vi "TestHTTP.vi"() -> ()   [LabVIEW 2025, in "MCP Server.lvlib"]
uses:
  MCP Server.lvlib
  MCP Handler/MCP Handler.lvclass
  C:/Program Files/National Instruments/LabVIEW 2025/vi.lib/IlluminatedG/IG HTTP Server/HTTP Server/Handler/Handler.lvclass
  <vilib>/IlluminatedG/IG HTTP Server/HTTP Server/Server/Add Connection Handler.vi
  <vilib>/IlluminatedG/IG HTTP Server/HTTP Server/Server/Add Request Handler.vi
  <vilib>/IlluminatedG/IG HTTP Server/HTTP Server/Server/Add Route Handler.vi
  <vilib>/IlluminatedG/IG HTTP Server/HTTP Server/Server/Add Controller Handler.vi
  <vilib>/IlluminatedG/IG HTTP Server/HTTP Server/Server/Add Controller.vi
  <vilib>/IlluminatedG/IG HTTP Server/HTTP Server/Server/Add Response Handler.vi
  <vilib>/IlluminatedG/IG HTTP Server/HTTP Server/Server/Add Complete Handler.vi
  <vilib>/IlluminatedG/IG HTTP Server/HTTP Server/Server/Add Exception Handler.vi
  <vilib>/IlluminatedG/IG HTTP Server/HTTP Server/Connection Handler/Connection Handler.lvclass
  <vilib>/IlluminatedG/IG HTTP Server/HTTP Server/Request Handler/Request Handler.lvclass
  <vilib>/IlluminatedG/IG HTTP Server/HTTP Server/Route Handler/Route Handler.lvclass
  <vilib>/IlluminatedG/IG HTTP Server/HTTP Server/Controller Handler/Controller Handler.lvclass
  <vilib>/IlluminatedG/IG HTTP Server/HTTP Server/Controller/Controller.lvclass
  <vilib>/IlluminatedG/IG HTTP Server/HTTP Server/Response Handler/Response Handler.lvclass
  <vilib>/IlluminatedG/IG HTTP Server/HTTP Server/Complete Handler/Complete Handler.lvclass
  <vilib>/IlluminatedG/IG HTTP Server/HTTP Server/Exception Handler/Exception Handler.lvclass
  <vilib>/IlluminatedG/IG HTTP Server/HTTP Server/Handler/Handler.lvclass
  C:/Program Files/National Instruments/LabVIEW 2025/vi.lib/IlluminatedG/IG HTTP Server/HTTP Server/Controller/Controller.lvclass
  C:/Users/jgoebel/OneDrive - Emerson/Dokumente/Praesentationen/MCP in LabVIEW/LabVIEW-MCP-Server-Toolkit/src/MCP Server/MCP Handler/MCP Handler.lvclass
  <vilib>/IlluminatedG/IG HTTP Server/HTTP Server/Server/Server.lvclass
panel:
  out "Numeric":i32
  in  "stop":bool
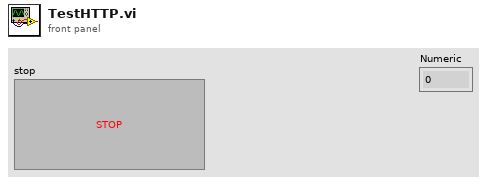
[diagram p1: front panel]
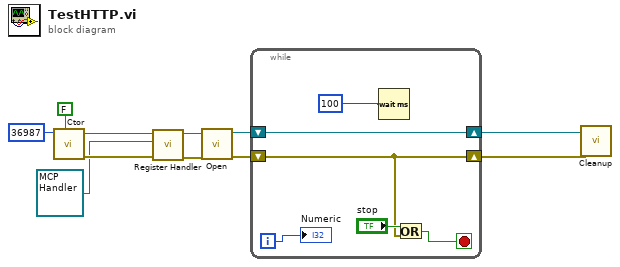
[diagram p0: block diagram]
diagram:
  n1 = call <vilib>:"Ctor.vi"("Debug (F)"=FALSE, "HTTP Port (80)"=u16 36987) -> ("error out"=w10:errorcluster, "Server out"=w11:refnum<class "Server.lvclass">)  [unwired: 8 in]
  n2 = call <vilib>:"Register Handler.vi"("error in (no error)"=w10, "Handler"=refnum<class "MCP Handler.lvclass"> refnum ("MCP Server.lvlib:MCP Handler.lvclass"), "Server in"=w11) -> ("error out"=w8:errorcluster, "Server out"=w9:refnum<class "Server.lvclass">)  [unwired: 7 in]
  n3 = call <vilib>:"Open.vi"("error in (no error)"=w8, "Server in"=w9) -> ("error out"=w6:errorcluster, "Server out"=w7:refnum<class "Server.lvclass">)  [unwired: 8 in]
  n4 = while {
    shift-right: [w12] -> w5
    shift-left: w6 -> [w12]
    shift-right: [w17] -> w4
    shift-left: w7 -> [w17]
    i -> [w14]
    stop <- w13 stop-if-true
    n5 = Wait (ms)(milliseconds to wait=u32 100) -> ()  [unwired: 1 out]
    n6 = Or(x="stop", y=w12) -> (x .or. y?=w13:bool)
    "Numeric" <- w14
  }
  n7 = call <vilib>:"Cleanup.vi"("error in (no error)"=w5, "Server in"=w4) -> ()  [unwired: 9 in, 1 out]
